vi "Variant Array to String Array.vi"(8 "error in (no error)":errorcluster, 11 "Variant":variant) -> (0 "error out":errorcluster, 3 "String Array":string[](array[string]))   [LabVIEW 2016, in "M1M3SupportEUI_Views.lvlib"]
uses:
  M1M3SupportEUI_Views.lvlib
  <vilib>/Utility/Data Type/NI_Data Type.lvlib
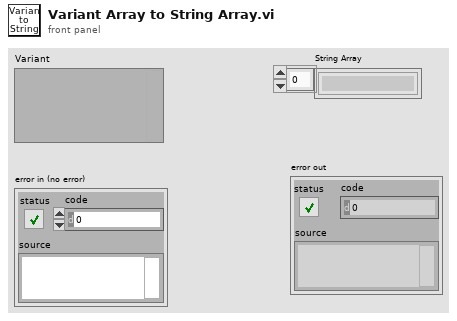
[diagram p1: front panel]
types:
  T1 = typedef "NI_Data Type.lvlib/Data Type.ctl" = enum8{"Invalid Type", "Void", "I8", "I16", "I32", "I64", "U8", "U16", "U32", "U64", "Single Float", "Double Float", "Extended Float", "Single Complex", "Double Complex", "Extended Complex", "Enum U8", "Enum U16", "Enum U32", "Enum U64", "Single Float With Unit", "Double Float With Unit", "Extended Float With Unit", "Single Complex with Unit", "Double Complex with Unit", "Extended Complex with Unit", "Boolean", "String", "Path", "Picture", "Tag", "Array", "Cluster", "Variant", "LV Variant", "Waveform", "Timestamp", "Digital Waveform", "Digital Data", "ExpressData", "Refnum", "External Data", "VI", "Poly VI", "LabVIEW Class Instance", "Fixed Point"}
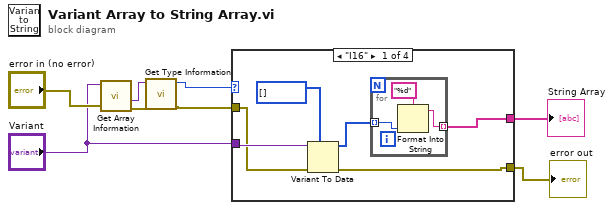
[diagram p0: block diagram]
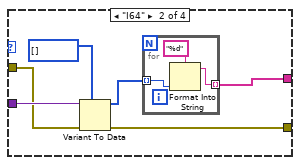
[diagram p2: hidden frame]
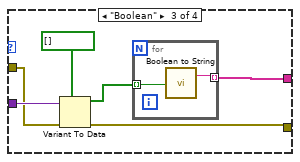
[diagram p3: hidden frame]
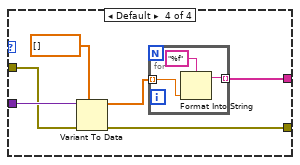
[diagram p4: hidden frame]
diagram:
  n1 = call <vilib>:"Get Array Information.vi"("error in (no error)"="error in (no error)", "Variant"="Variant") -> ("error out"=w5:errorcluster, "Array Element Data Type"=w6:variant)  [unwired: 6 in, 2 out]
  n2 = call <vilib>:"Get Type Information.vi"("error in (no error)"=w5, "Variant"=w6) -> ("error out"=w8:errorcluster, "Type"=w7:T1)  [unwired: 5 in, 3 out]
  n3 = case shown="\"I16\"" w7 {
    tunnel: "Variant" -> [w13 w21 w31 w40]
    tunnel: [w9 w18 w27 w36] -> w3
    tunnel: w8 -> [w12 w20 w30 w38]
    tunnel: [w11 w19 w29 w35] -> w2
    frame "I16" {
      n4 = Variant To Data(error in=w12, type=i16[] [], Variant=w13) -> (data=w10:i16[], error out=w11:errorcluster)
      n5 = for {
        tunnel: w10 -> [w17] mode=indexing
        tunnel: [w16] -> w9 mode=indexing
        n6 = Format Into String(format string="%d", w17) -> (resulting string=w16:string)  [unwired: 2 in, 1 out]
      }
    }
    frame "I64" {
      n7 = Variant To Data(error in=w20, type=i64[] [], Variant=w21) -> (data=w22:i64[], error out=w19:errorcluster)
      n8 = for {
        tunnel: w22 -> [w26] mode=indexing
        tunnel: [w25] -> w18 mode=indexing
        n9 = Format Into String(format string="%d", w26) -> (resulting string=w25:string)  [unwired: 2 in, 1 out]
      }
    }
    frame "Boolean" {
      n10 = Variant To Data(error in=w30, type=bool[] [], Variant=w31) -> (data=w28:bool[], error out=w29:errorcluster)
      n11 = for {
        tunnel: w28 -> [w34] mode=indexing
        tunnel: [w33] -> w27 mode=indexing
        n12 = call "Boolean to String.vi"("BooleanValue"=w34) -> ("StringForm"=w33:string)  [unwired: 1 out]
      }
    }
    frame Default {
      n13 = Variant To Data(error in=w38, type=sgl[] [], Variant=w40) -> (data=w37:sgl[], error out=w35:errorcluster)
      n14 = for {
        tunnel: w37 -> [w43] mode=indexing
        tunnel: [w42] -> w36 mode=indexing
        n15 = Format Into String(format string="%f", w43) -> (resulting string=w42:string)  [unwired: 2 in, 1 out]
      }
    }
  }
  "String Array" <- w3
  "error out" <- w2
